vi "Facade.vi"(0 "Data In":T4, 2 "Display State In":T2, 3 "Container State":T3) -> (6 "Data Out":T4, 7 "Display State Out":T2, 8 "Action":T1)   [LabVIEW 2015, in "KRing.xctl"]
uses:
  KRing.xctl
  Data.ctl
  <vilib>/_xctls/Container State.ctl
  State.ctl
  <vilib>/_xctls/Action.ctl
  <vilib>/_xctls/XControlSupport.lvlib
panel:
  in  "Ring":u16(ring)
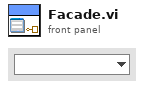
[diagram p1: front panel]
types:
  T1 = typedef "XControlSupport.lvlib/Action.ctl" = cluster{"Data Changed?":bool, "State Changed?":bool, "Action Name":string}
  T2 = typedef "KRing.xctl/State.ctl" = cluster{"mixed":bool, "Value":i16, "Ring":refnum<vi>}
  T3 = typedef "XControlSupport.lvlib/Container State.ctl" = cluster{"Indicator?":bool, "Run Mode?":bool, " Refnum":refnum<vi>}
  T4 = typedef "KRing.xctl/Data.ctl" = i16
  T5 = typedef "LVStringsAndValuesArrayTypeDef_U16.ctl" = cluster{"String":string, "Value":u16}[]
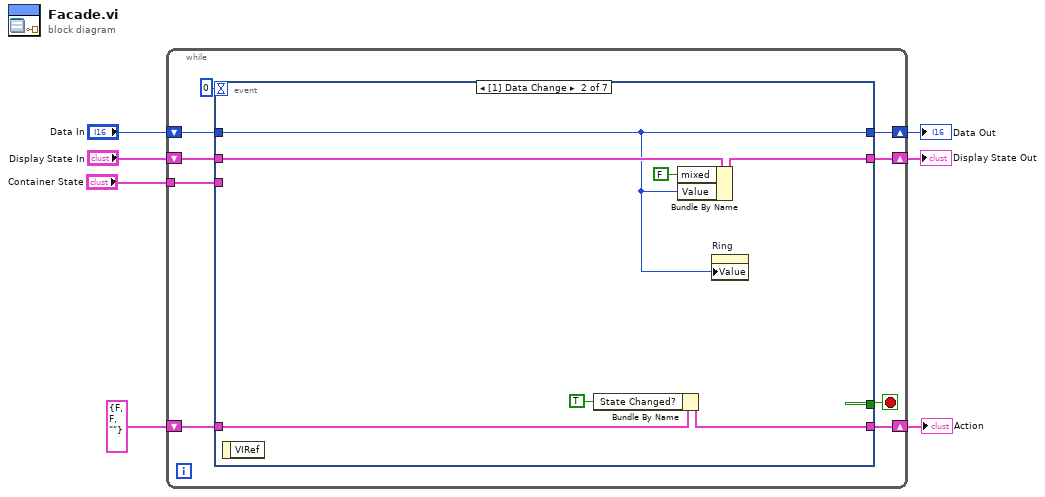
[diagram p0: block diagram]
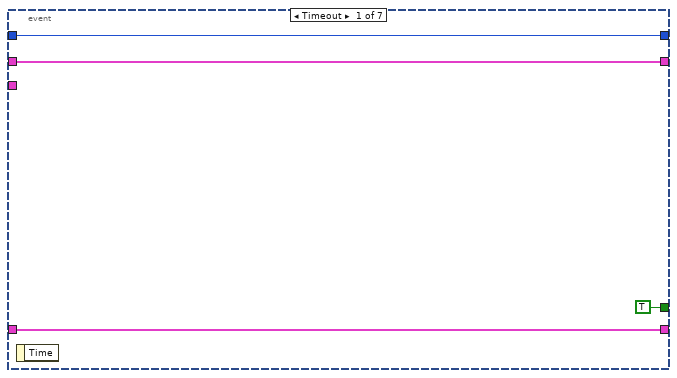
[diagram p2: hidden frame]
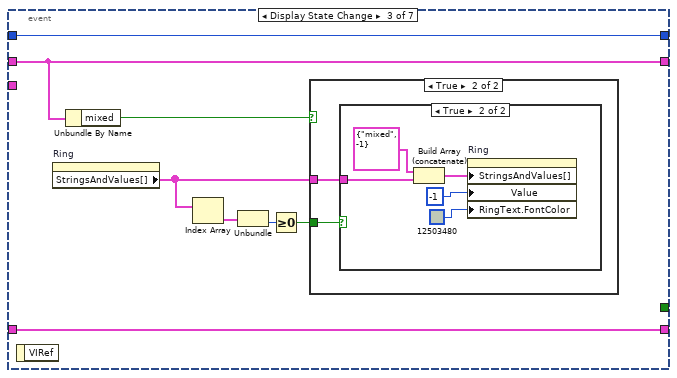
[diagram p3: hidden frame]
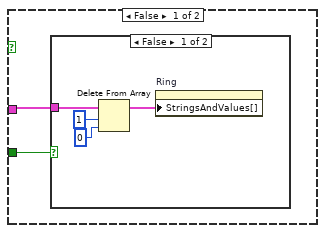
[diagram p4: hidden frame]
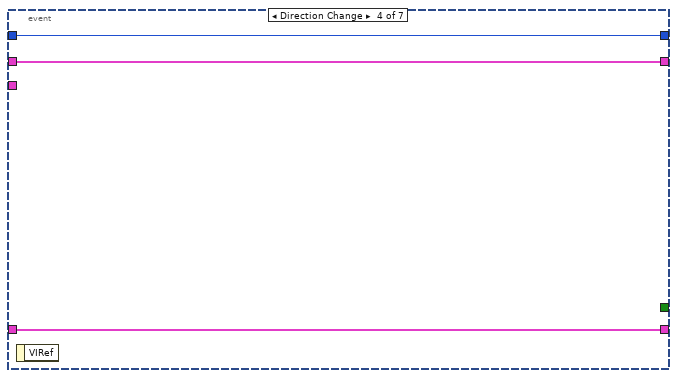
[diagram p7: hidden frame]
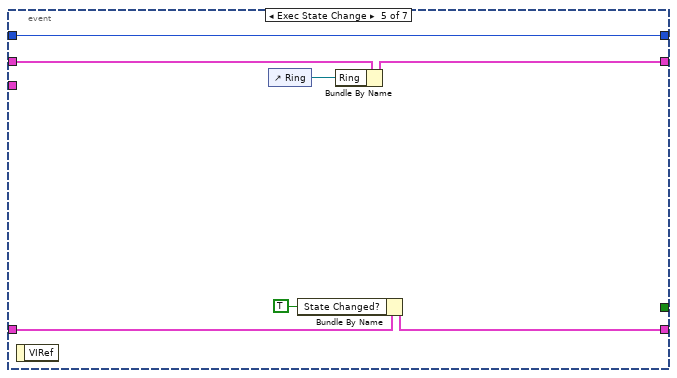
[diagram p8: hidden frame]
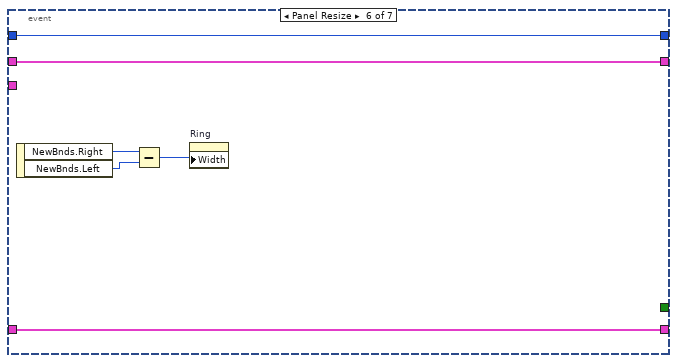
[diagram p9: hidden frame]
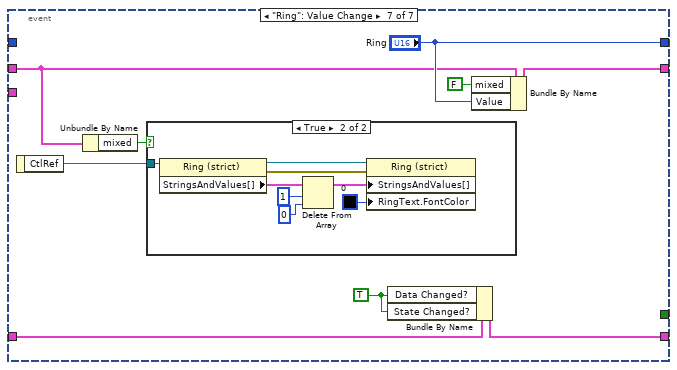
[diagram p10: hidden frame]
diagram:
  n1 = while {
    shift-right: [w15] -> w4
    shift-left: "Display State In" -> [w16]
    tunnel: "Container State" -> [w12]
    shift-right: [w10] -> w7
    shift-left: "Data In" -> [w11]
    shift-right: [w8] -> w2
    shift-left: T1 {"Data Changed?"=FALSE, "State Changed?"=FALSE, "Action Name"=""} ("Action") -> [w9]
    stop <- w14 stop-if-true
    n2 = event shown="[1] Data Change" {
      selector: _ -> [_ _ _ _ _ _ _]
      dyn-events: _ -> [_ _ _ _ _ _ _]
      timeout: 0 -> [_ _ _ _ _ _ _]
      tunnel: w16 -> [w18 w27 w33 w51 w58 w64 w68]
      tunnel: [w18 w25 w33 w51 w55 w64 w72] -> w15
      tunnel: [TRUE _ _ _ _ _ _] -> w14
      tunnel: w12 -> [_ _ _ _ _ _ _]
      tunnel: w11 -> [w17 w21 w35 w50 w57 w63 _]
      tunnel: [w17 w21 w35 w50 w57 w63 "Ring"] -> w10
      tunnel: [w19 w23 w34 w49 w53 w62 w70] -> w8
      tunnel: w9 -> [w19 w26 w34 w49 w56 w62 w73]
      event Timeout {
        n3 = event-data() -> ()  [unwired: 1 in, 1 out]
      }
      event Data Change {
        n4 = event-data() -> ()  [unwired: 1 in, 1 out]
        n5 = Bundle By Name(cluster=w26, "State Changed?"=TRUE) -> (w23:T1)
        n6 = Bundle By Name(cluster=w27, "mixed"=FALSE, "Value"=w21) -> (w25:T2)
        n7 = property on="Ring" class="Ring (strict)"("Value"=w21) -> ()  [unwired: 2 in, 2 out]
      }
      event Display State Change {
        n8 = event-data() -> ()  [unwired: 1 in, 1 out]
        n9 = property on="Ring" class="Ring (strict)"() -> ("StringsAndValues[]"=w28:T5)  [unwired: 2 in, 2 out]
        n10 = Unbundle By Name(w33) -> ("mixed"=w31:bool)
        n11 = Index Array(array=w28) -> (element=w32:cluster{"String":string, "Value":u16})  [unwired: 1 in]
        n12 = Unbundle(w32) -> ("Value"=w30:u16)  [unwired: 1 out]
        n13 = Greater Or Equal To 0?(x=w30) -> (x >= 0?=w29:bool)
        n14 = case shown="True" w31 {
          tunnel: w29 -> [w37 w43]
          tunnel: w28 -> [w36 w42]
          frame False {
            n15 = case shown="False" w37 {
              tunnel: w36 -> [w41 _]
              frame False {
                n16 = Delete From Array(array=w41, length=1, index=0) -> (array with subset deleted=w38:T5)  [unwired: 1 out]
                n17 = property on="Ring" class="Ring (strict)"("StringsAndValues[]"=w38) -> ()  [unwired: 2 in, 2 out]
              }
              frame True {
              }
            }
          }
          frame True {
            n18 = case shown="True" w43 {
              tunnel: w42 -> [_ w48]
              frame False {
              }
              frame True {
                n19 = Build Array (concatenate)(cluster{"String":string, "Value":i16} {"String"="mixed", "Value"=-1} ("element"), w48) -> (w46:T5)
                n20 = property on="Ring" class="Ring (strict)"("StringsAndValues[]"=w46, "Value"=i16 -1, "RingText.FontColor"=u32 12503480) -> ()  [unwired: 2 in, 2 out]
              }
            }
          }
        }
      }
      event Direction Change {
        n21 = event-data() -> ()  [unwired: 1 in, 1 out]
      }
      event Exec State Change {
        n22 = event-data() -> ()  [unwired: 1 in, 1 out]
        n23 = control-ref of="Ring"() -> (w54:refnum<vi>)
        n24 = Bundle By Name(cluster=w56, "State Changed?"=TRUE) -> (w53:T1)
        n25 = Bundle By Name(cluster=w58, "Ring"=w54) -> (w55:T2)
      }
      event Panel Resize {
        n26 = event-data() -> ("NewBnds.Right"=w61:i16, "NewBnds.Left"=w60:i16)  [unwired: 1 in]
        n27 = Subtract(x=w61, y=w60) -> (x-y=w59:i16)
        n28 = property on="Ring" class="Ring (strict)"("Width"=w59) -> ()  [unwired: 2 in, 2 out]
      }
      event "Ring": Value Change {
        w65 = TRUE ("State Changed?")
        n29 = event-data() -> ("CtlRef"=w66:refnum<vi>)  [unwired: 1 in]
        n30 = Unbundle By Name(w68) -> ("mixed"=w67:bool)
        n31 = case shown="True" w67 {
          tunnel: w66 -> [_ w77]
          frame False {
          }
          frame True {
            n32 = property on="Property Node" class="Ring (strict)"(reference=w77) -> (reference out=w76:refnum<vi>, error out=w75:errorcluster, "StringsAndValues[]"=w78:T5)  [unwired: 1 in]
            n33 = Delete From Array(array=w78, length=1, index=0) -> (array with subset deleted=w81:T5)  [unwired: 1 out]
            n34 = property on="Property Node" class="Ring (strict)"(reference=w76, error in=w75, "StringsAndValues[]"=w81, "RingText.FontColor"=u32 0) -> ()  [unwired: 2 out]
          }
        }
        n35 = Bundle By Name(cluster=w73, "Data Changed?"=w65, "State Changed?"=w65) -> (w70:T1)
        n36 = Bundle By Name(cluster=w68, "mixed"=FALSE, "Value"="Ring") -> (w72:T2)
      }
    }
  }
  "Display State Out" <- w4
  "Data Out" <- w7
  "Action" <- w2
